vi "Get Ext Trigger Mode.vi"(7 "Ref Trigger Mode":refnum<vi>, 8 "error in":errorcluster, 10 "Pulsar Handle":i16, 11 "OphirFastX (in)":refnum<k7>) -> (0 "error out":errorcluster, 3 "OphirFastX (out)":refnum<k7>)   [LabVIEW 2009]
panel:
  # "Guillaume Plateau - yguig2@yahoo.fr"
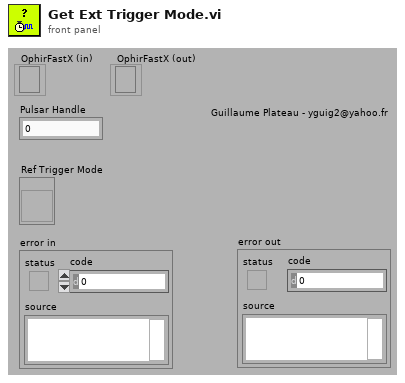
[diagram p1: front panel]
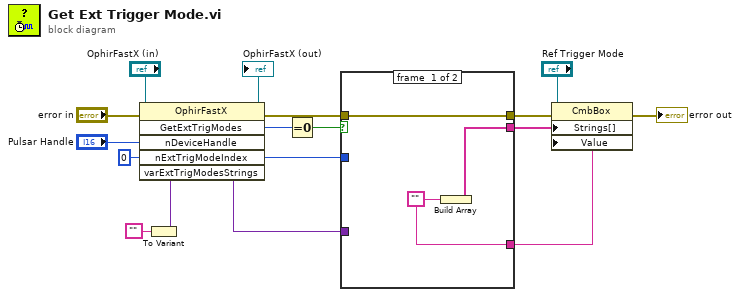
[diagram p0: block diagram]
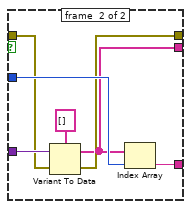
[diagram p2: hidden frame]
diagram:
  n1 = To Variant(anything="") -> (Variant=w5:variant)
  n2 = invoke class="OphirFastX" method="GetExtTrigModes"(reference="OphirFastX (in)", error in="error in", "nDeviceHandle"="Pulsar Handle", "nExtTrigModeIndex"=i16 0, "varExtTrigModesStrings"=w5) -> (reference out=→"OphirFastX (out)":refnum<k7>, error out=w15:errorcluster, "GetExtTrigModes"=w13:i32, "nExtTrigModeIndex"=w3:i16, "varExtTrigModesStrings"=w4:variant)  [unwired: 1 in, 1 out]
  n3 = Equal To 0?(x=w13) -> (x = 0?=w14:bool)
  n4 = case shown="True" w14 {
    tunnel: w4 -> [_ w27]
    tunnel: w15 -> [w19 w24]
    tunnel: [w18 w21] -> w6
    tunnel: [w20 w23] -> w8
    tunnel: [w19 w22] -> w10
    tunnel: w3 -> [_ w25]
    frame #0 {
      w20 = ""
      n5 = Build Array(w20) -> (w18:string[])
    }
    frame #1 {
      n6 = Variant To Data(error in=w24, Variant=w27, type=string[] []) -> (error out=w22:errorcluster, data=w21:string[])
      n7 = Index Array(array=w21, index=w25) -> (element=w23:string)
    }
  }
  n8 = property class="CmbBox"(reference="Ref Trigger Mode", error in=w10, "Strings[]"=w6, "Value"=w8) -> (error out=→"error out":errorcluster)  [unwired: 1 out]
